vi "dfd_Util Convert I32 to I160.vi"(2 "x [I32]":i32) -> (7 "x [I160]":T1)   [LabVIEW 2017, in "NI_DigFilter_FXP.lvlib"]
uses:
  <vilib>/addons/Digital Filter Design/NI_DigFilter_FXP.lvlib
  <vilib>/addons/Digital Filter Design/_Objects.llb/dfd_Integer I160.ctl
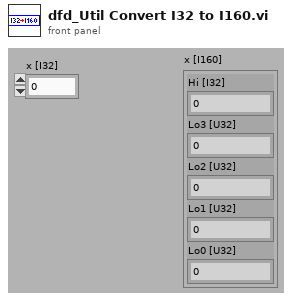
[diagram p1: front panel]
types:
  T1 = typedef "dfd_Integer I160.ctl" = cluster{"Hi [I32]":i32, "Lo3 [U32]":u32, "Lo2 [U32]":u32, "Lo1 [U32]":u32, "Lo0 [U32]":u32}
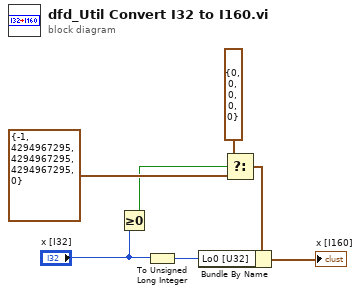
[diagram p0: block diagram]
diagram:
  n1 = Greater Or Equal To 0?(x="x [I32]") -> (x >= 0?=w1:bool)
  n2 = To Unsigned Long Integer(number="x [I32]") -> (unsigned 32bit integer=w2:u32)
  n3 = Select(t=T1 {"Hi [I32]"=0, "Lo3 [U32]"=0, "Lo2 [U32]"=0, "Lo1 [U32]"=0, "Lo0 [U32]"=0} ("x"), s=w1, f=T1 {"Hi [I32]"=-1, "Lo3 [U32]"=4294967295, "Lo2 [U32]"=4294967295, "Lo1 [U32]"=4294967295, "Lo0 [U32]"=0} ("x")) -> (s? t:f=w4:T1)
  n4 = Bundle By Name(cluster=w4, "Lo0 [U32]"=w2) -> (→"x [I160]":T1)
